vi "Page_Advanced_Write.vi"(6 "ctlReferences":T1, 8 "error in (no error)":errorcluster, 11 "Class in":refnum<class "Installer.lvclass">) -> (0 "error out":errorcluster, 3 "Class out":refnum<class "Installer.lvclass">)   [LabVIEW 2020, in "Installer.lvclass"]
uses:
  <vilib>/AppBuilder/IB_Classes/Installer/Installer.lvclass
  <vilib>/AppBuilder/IB_Classes/Installer/Installer.lvclass/Installer.ctl
  <resource>/Framework/Providers/Builds/Installer/Pages/controls/IB_UI_Page_Advanced_References.ctl
  <resource>/Framework/Providers/Builds/Installer/CDK_sTypeDef_SystemRequirements.ctl
  <resource>/Framework/Providers/Common/provcom_BrowseProjectFile2.ctl
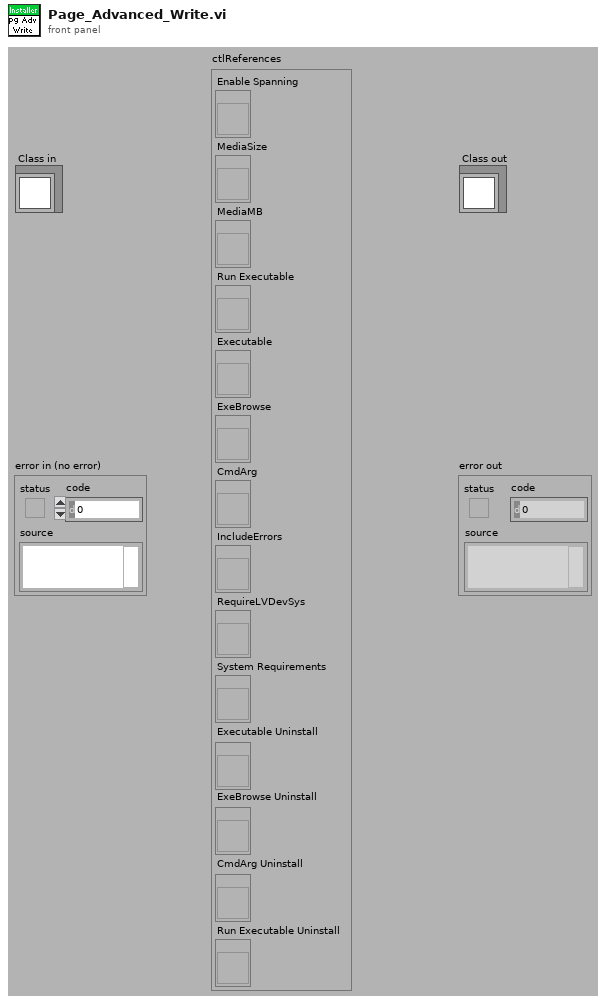
[diagram p1: front panel]
types:
  T1 = typedef "IB_UI_Page_Advanced_References.ctl" = cluster{"Enable Spanning":refnum<vi>, "MediaSize":refnum<vi>, "MediaMB":refnum<vi>, "Run Executable":refnum<vi>, "Executable":refnum<vi>, "ExeBrowse":refnum<vi>, "CmdArg":refnum<vi>, "IncludeErrors":refnum<vi>, "RequireLVDevSys":refnum<vi>, "System Requirements":refnum<vi>, "Executable Uninstall":refnum<vi>, "ExeBrowse Uninstall":refnum<vi>, "CmdArg Uninstall":refnum<vi>, "Run Executable Uninstall":refnum<vi>}
  T2 = typedef "IB_Installer.ctl" = cluster{"Destination":refnum<class "IB_Destination.lvclass">[], "Source":refnum<class "IB_Source.lvclass">[], "buildObject":T3, "defaultDir":string, "platform":string, "author":string, "productName":string, "buildSpecName":string, "hide":bool, "requireLVDevSys":bool, "autoIncrement":bool, "includeError":bool, "readmeID":string, "buildLocation":path, "readmePath":path, "mediaSize":u16, "language":T4, "productVersion":T5, "preview":bool, "programmatic":bool, "progressBarEvents":T6, "userLog_Path":path, "shortcutAddresses":T8[], "EXE_Install Address":string, "EXE_Uninstall Address":string, "additional NIPaths":refnum<class "Dest_NI_NIPath.lvclass">[], "web service itemIDs":string[], "installerName":string}
  T3 = typedef "ItemRef.ctl" = u64
  T4 = typedef "CDK_sTypeDef_Languages.ctl" = u16
  T5 = typedef "CDK_sTypeDef_ProductVersion.ctl" = cluster{"Major":u8, "Minor":u8, "Update":u16}
  T6 = typedef "provcom_ProgressBar_Events.ctl" = cluster{"newJob":refnum<user-event>, "newItem":refnum<user-event>, "errorMsg":T7, "cancel":refnum<user-event>}
  T7 = typedef "mxLvBuildError.ctl" = refnum<user-event>
  T8 = typedef "CDK_sTypeDef_ShortcutAddress.ctl" = cluster{"file":string, "shortcut":string}
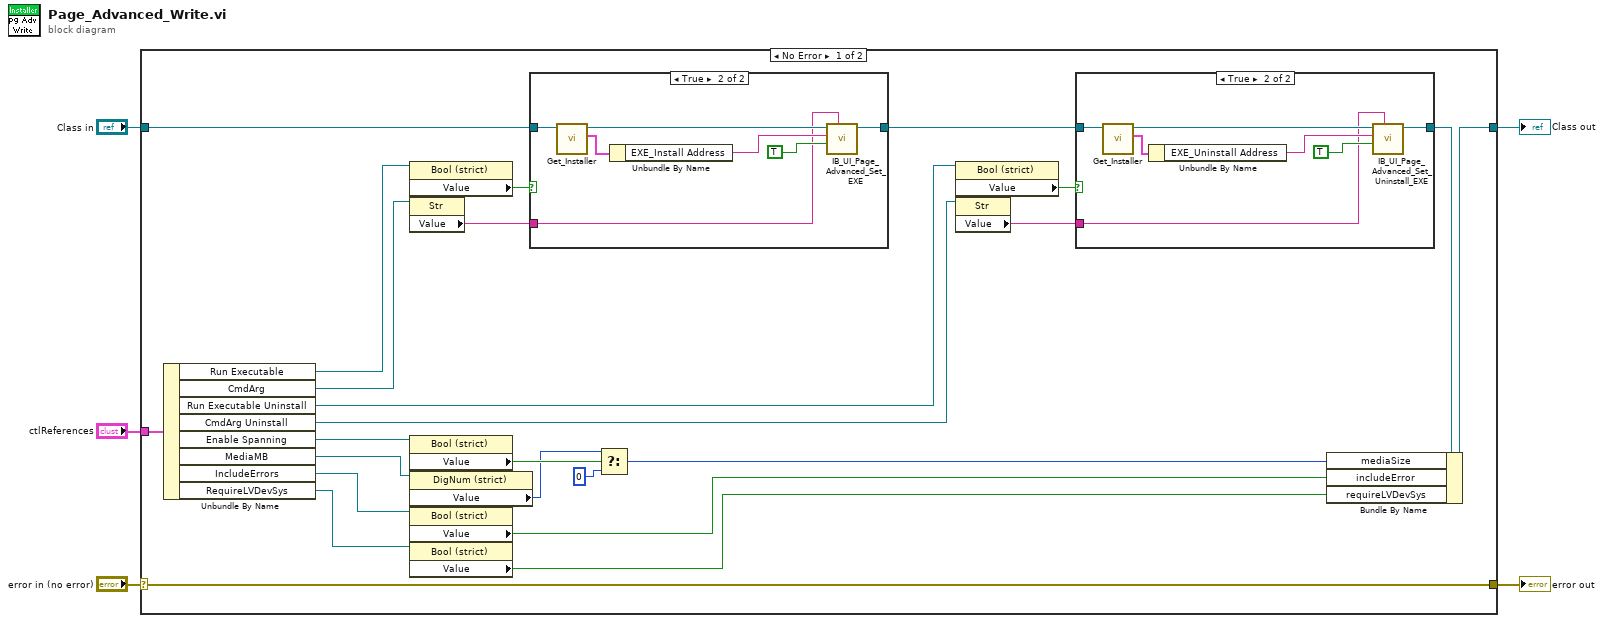
[diagram p0: block diagram]
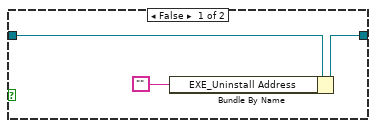
[diagram p2: hidden frame]
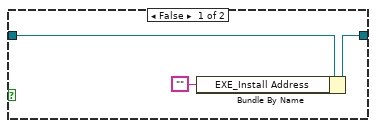
[diagram p3: hidden frame]
diagram:
  n1 = case shown="No Error" "error in (no error)" {
    selector: "error in (no error)" -> [w27 w51]
    tunnel: [w27 w51] -> w4
    tunnel: [w28 w50] -> w2
    tunnel: "Class in" -> [w15 w50]
    tunnel: "ctlReferences" -> [w29 _]
    frame No Error {
      n2 = Unbundle By Name(w29) -> ("Run Executable"=w14:refnum<vi>, "CmdArg"=w13:refnum<vi>, "Run Executable Uninstall"=w9:refnum<vi>, "CmdArg Uninstall"=w8:refnum<vi>, "Enable Spanning"=w26:refnum<vi>, "MediaMB"=w25:refnum<vi>, "IncludeErrors"=w24:refnum<vi>, "RequireLVDevSys"=w23:refnum<vi>)
      n3 = property class="Bool (strict)"(reference=w14) -> ("Value"=w16:bool)  [unwired: 1 in, 2 out]
      n4 = property class="Str"(reference=w13) -> ("Value"=w12:string)  [unwired: 1 in, 2 out]
      n5 = property class="Bool (strict)"(reference=w26) -> ("Value"=w19:bool)  [unwired: 1 in, 2 out]
      n6 = property class="DigNum (strict)"(reference=w25) -> ("Value"=w17:u16)  [unwired: 1 in, 2 out]
      n7 = property class="Bool (strict)"(reference=w24) -> ("Value"=w22:bool)  [unwired: 1 in, 2 out]
      n8 = property class="Bool (strict)"(reference=w23) -> ("Value"=w21:bool)  [unwired: 1 in, 2 out]
      n9 = case shown="True" w16 {
        tunnel: w15 -> [w42 w45]
        tunnel: [w41 w43] -> w7
        tunnel: w12 -> [_ w44]
        frame False {
          n10 = Bundle By Name(cluster=w42, "EXE_Install Address"="") -> (w41:refnum<class "Installer.lvclass">)
        }
        frame True {
          n11 = call <vilib>:"Get_Installer.vi"("Installer in"=w45) -> ("data"=w47:T2, "Installer out"=w49:refnum<class "Installer.lvclass">)  [unwired: 1 in, 8 out]
          n12 = Unbundle By Name(w47) -> ("EXE_Install Address"=w48:string)
          n13 = call <resource>:"IB_UI_Page_Advanced_Set_EXE.vi"("cmdArg"=w44, "runEXE"=TRUE, "address"=w48, "Installer in"=w49) -> ("Installer out"=w43:refnum<class "Installer.lvclass">)  [unwired: 2 in, 5 out]
        }
      }
      n14 = Select(t=w17, s=w19, f=u16 0) -> (s? t:f=w18:u16)
      n15 = property class="Bool (strict)"(reference=w9) -> ("Value"=w10:bool)  [unwired: 1 in, 2 out]
      n16 = property class="Str"(reference=w8) -> ("Value"=w11:string)  [unwired: 1 in, 2 out]
      n17 = case shown="True" w10 {
        tunnel: [w32 w34] -> w6
        tunnel: w11 -> [_ w35]
        tunnel: w7 -> [w30 w33]
        frame False {
          n18 = Bundle By Name(cluster=w30, "EXE_Uninstall Address"="") -> (w32:refnum<class "Installer.lvclass">)
        }
        frame True {
          n19 = call <vilib>:"Get_Installer.vi"("Installer in"=w33) -> ("data"=w37:T2, "Installer out"=w39:refnum<class "Installer.lvclass">)  [unwired: 1 in, 8 out]
          n20 = Unbundle By Name(w37) -> ("EXE_Uninstall Address"=w38:string)
          n21 = call <resource>:"IB_UI_Page_Advanced_Set_Uninstall_EXE.vi"("CmdArg_Uninstall"=w35, "EXE_Uninstall"=TRUE ("runEXE"), "address"=w38, "Installer in"=w39) -> ("Installer out"=w34:refnum<class "Installer.lvclass">)  [unwired: 6 in, 1 out]
        }
      }
      n22 = Bundle By Name(cluster=w6, "mediaSize"=w18, "includeError"=w22, "requireLVDevSys"=w21) -> (w28:refnum<class "Installer.lvclass">)
    }
    frame Error {
    }
  }
  "error out" <- w4
  "Class out" <- w2
